vi "Collect Data.vi"(8 "error in (no error)":errorcluster, 10 "AbstractData in":refnum<class "AbstractData.lvclass">, 11 "AbstractCollector1D in":refnum<class "AbstractCollector1D.lvclass">) -> (0 "error out":errorcluster, 2 "finished?":bool=TRUE, 3 "AbstractCollector1D out":refnum<class "AbstractCollector1D.lvclass">)   [LabVIEW 2014, in "AbstractCollector1D.lvclass"]
uses:
  AbstractCollector1D.lvclass
  Model/Data/AbstractData/AbstractData.lvclass
  Model/Data/Data1D/Data1D.lvclass
  Data1D Cluster.ctl
  AbstractCollector/AbstractCollector.lvclass
  Interfaces/Observable Actor/Observable Actor.lvclass
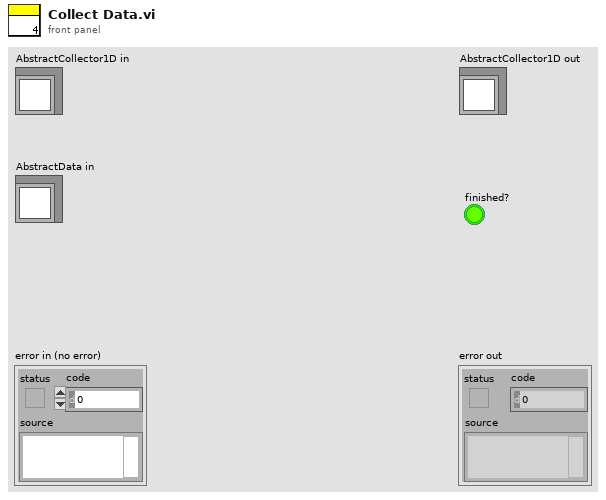
[diagram p1: front panel]
types:
  T1 = typedef "AbstractCollector1D.lvclass/Data1D Cluster.ctl" = cluster{"in":refnum<class "Data1D.lvclass">, "intermediate":refnum<class "Data1D.lvclass">}
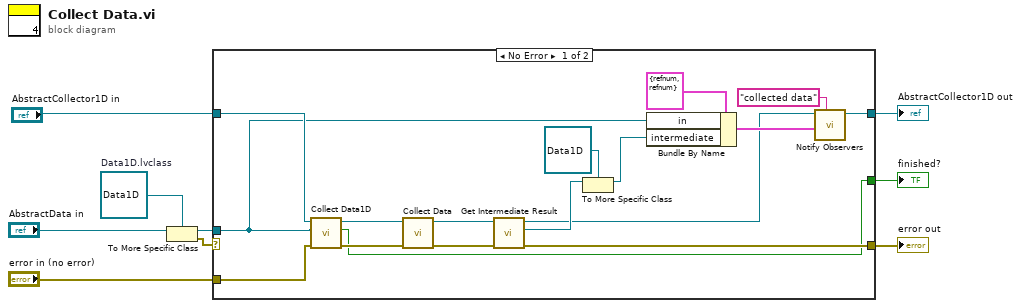
[diagram p0: block diagram]
diagram:
  w8 = refnum<class "Data1D.lvclass"> refnum  # Data1D.lvclass
  n1 = To More Specific Class(target class=w8, reference="AbstractData in") -> (specific class reference=w6:refnum<class "Data1D.lvclass">, error out=w7:errorcluster)  [unwired: 1 in]
  n2 = case shown="No Error" w7 {
    tunnel: w6 -> [w11 _]
    tunnel: "error in (no error)" -> [w10 w28]
    tunnel: [w20 w28] -> w4
    tunnel: "AbstractCollector1D in" -> [w12 w27]
    tunnel: [w22 w27] -> w2
    tunnel: [w15 _] -> w1
    frame No Error {
      n3 = call-dynamic "Collect Data1D.vi"("error in (no error)"=w10, "Data1D in"=w11, "AbstractCollector1D in"=w12) -> ("error out"=w16:errorcluster, "finished?"=w15:bool, "AbstractCollector1D out"=w17:refnum<class "AbstractCollector1D.lvclass">)  [unwired: 6 in]
      n4 = call-parent "Collect Data.vi"("error in (no error)"=w16, "AbstractCollector in"=w17) -> ("error out"=w13:errorcluster, "AbstractCollector out"=w14:refnum<class "AbstractCollector1D.lvclass">)  [unwired: 7 in, 1 out]
      n5 = call-dynamic "Get Intermediate Result.vi"("error in (no error)"=w13, "AbstractCollector in"=w14) -> ("error out"=w20:errorcluster, "AbstractData.lvclass"=w25:refnum<class "AbstractData.lvclass">, "AbstractCollector out"=w19:refnum<class "AbstractCollector1D.lvclass">)  [unwired: 7 in]
      n6 = To More Specific Class(target class=refnum<class "Data1D.lvclass"> refnum ("Data1D.lvclass"), reference=w25) -> (specific class reference=w23:refnum<class "Data1D.lvclass">)  [unwired: 1 in, 1 out]
      n7 = Bundle By Name(cluster=T1 {"in"=refnum, "intermediate"=refnum} ("Cluster"), "in"=w11, "intermediate"=w23) -> (w21:T1)
      n8 = call "Notify Observers.vi"("name"="collected data", "value"=w21, "Observable Actor in"=w19) -> ("Observable Actor out"=w22:refnum<class "AbstractCollector1D.lvclass">)  [unwired: 7 in, 1 out]
    }
    frame Error {
    }
  }
  "error out" <- w4
  "AbstractCollector1D out" <- w2
  "finished?" <- w1
